vi "ConnectionStatusName.vi"() -> (1 "message name":string)   [LabVIEW 2017, in "ServerComm.lvlib"]
doc: "Returns the following message name: ServerComm.ConnectionStatus. Subscribe to this message to receive updates when the connection between the device and NI InsightCM Server changes status. The NI-developed Server Comm process sends ServerComm.ConnectionStatus messages."
uses:
  <vilib>/addons/InsightCM/Devices/Shared/Common/ServerComm/ServerComm.lvlib
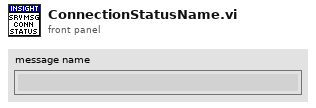
[diagram p1: front panel]
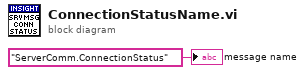
[diagram p0: block diagram]
diagram:
  "message name" <- "ServerComm.ConnectionStatus" ("ProcessName")
